vi "Normal to Backslash Codes String.vi"(11 "Normal String in":string) -> (3 "Backslash String out":string)   [LabVIEW 2018, in "String Data Type.lvclass"]
uses:
  String Data Type.lvclass
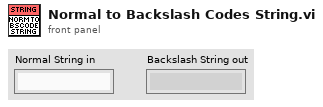
[diagram p1: front panel]
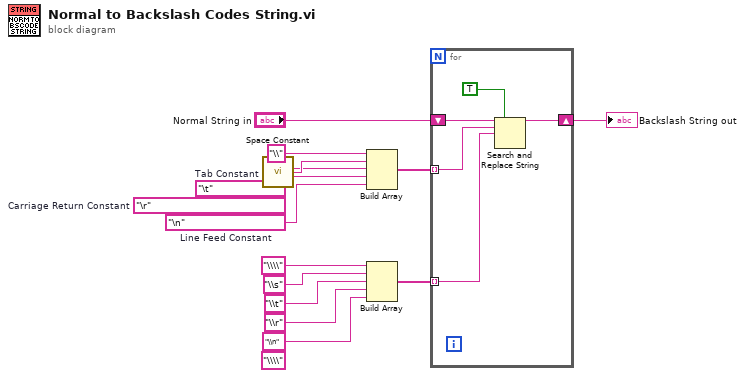
[diagram p0: block diagram]
diagram:
  (unwired) "\\\\"
  w10 = "\n"  # Line Feed Constant
  w11 = "\r"  # Carriage Return Constant
  w12 = "\t"  # Tab Constant
  n1 = call <vilib>:"Space Constant.vi"() -> ("String"=w13:string)
  n2 = Build Array("\\", w13, w12, w11, w10) -> (w9:string[])
  n3 = Build Array("\\\\", "\\s", "\\t", "\\r", "\\n") -> (w3:string[])
  n4 = for {
    tunnel: w9 -> [w18] mode=indexing
    tunnel: w3 -> [w17] mode=indexing
    shift-right: [w16] -> w1
    shift-left: "Normal String in" -> [w19]
    n5 = Search and Replace String(replace all?=TRUE ("replace all? (F)"), input string=w19, search string=w18, replace string=w17) -> (result string=w16:string)  [unwired: 4 in, 3 out]
  }
  "Backslash String out" <- w1
